vi "Caja fuerte No muerta.vi"() -> ()   [LabVIEW 2022 SP3]
doc: "Mi caja fuerte por Vess:3\n\nsimula el movimiento de una caja fuerte a la cual hay que darle una combinación y ya con esta saber\nsi la combinación es correcta o mala y después usar producto consumidor para enlistar los datos que van\na ser los movimientos que se harán para simular que la perilla gire"
panel:
  in  "Manija":i32(knob) min=0 max=100 step=1 scale=0.0..30.0
  out "Mensaje":string
  out "Arreglo C.":i32[](array[numeric])
  in  "Reinicio":bool
  in  "Enum":T1(ring)
  in  "stop":bool
  # "Combinación:\n11-7-10-21"
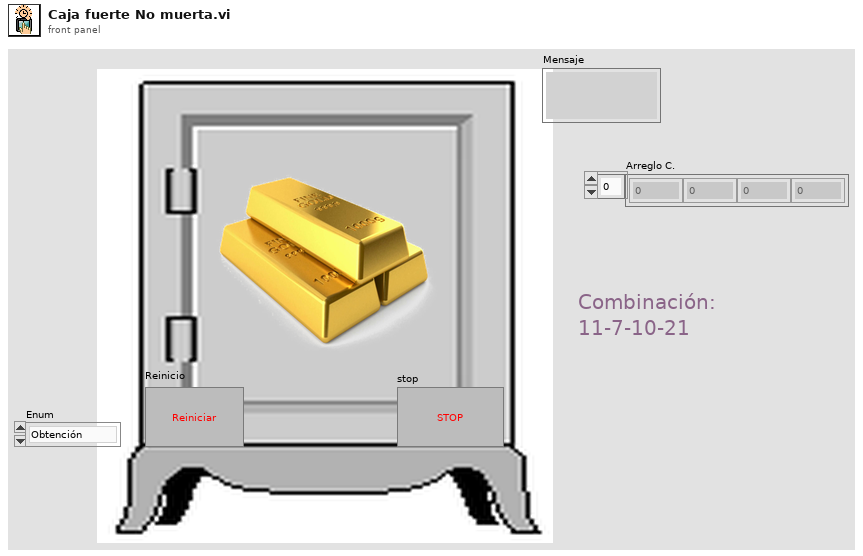
[diagram p1: front panel]
types:
  T1 = enum16{"Obtención", "Comprobación", "Fallo ", "Logro"}
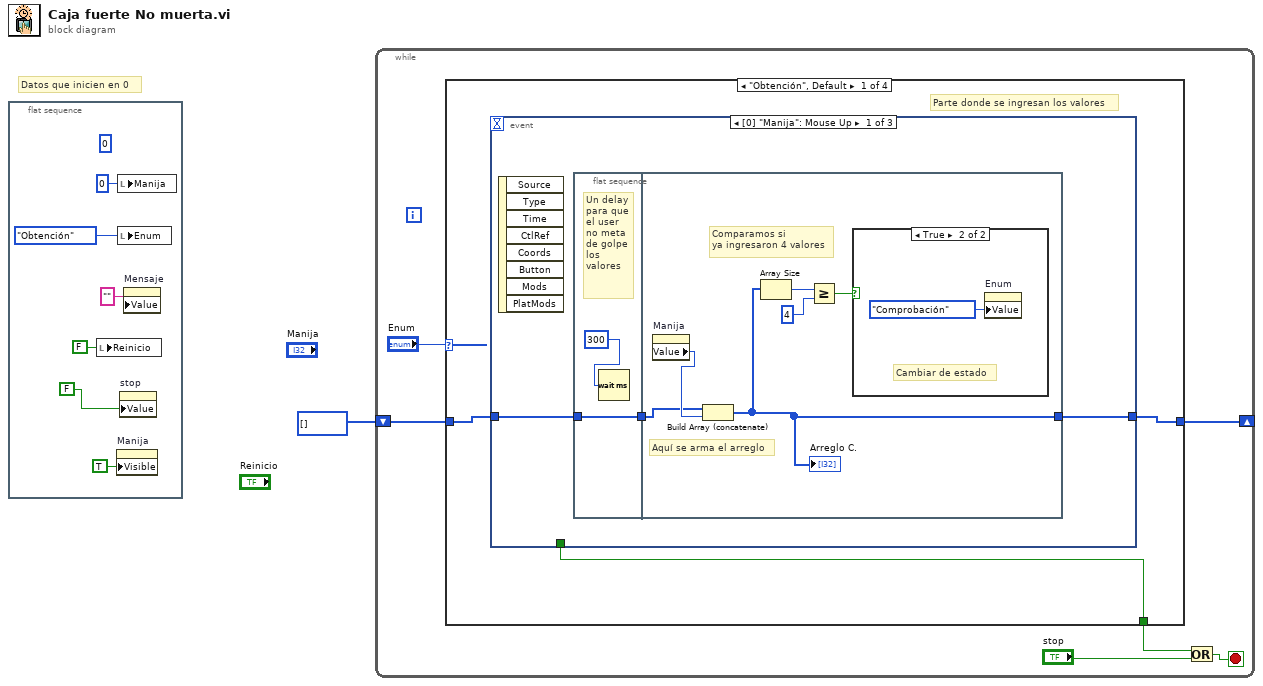
[diagram p0: block diagram]
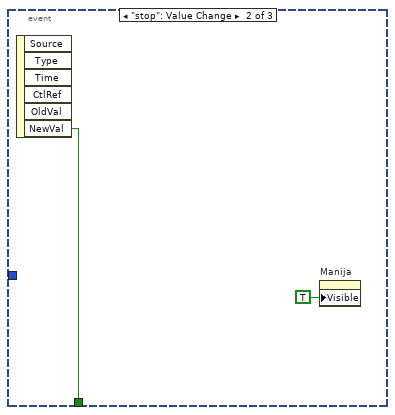
[diagram p3: hidden frame]
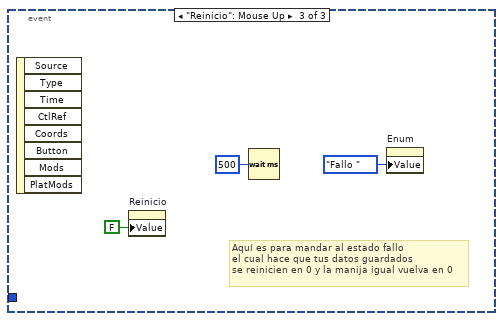
[diagram p4: hidden frame]
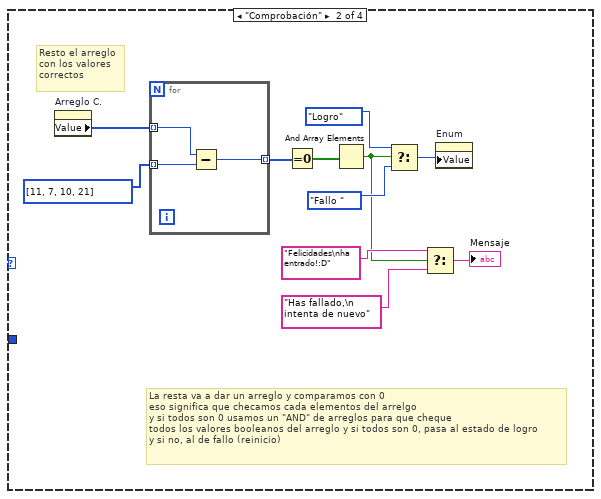
[diagram p5: hidden frame]
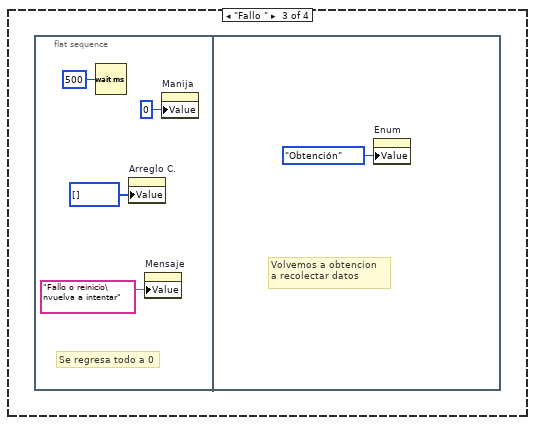
[diagram p6: hidden frame]
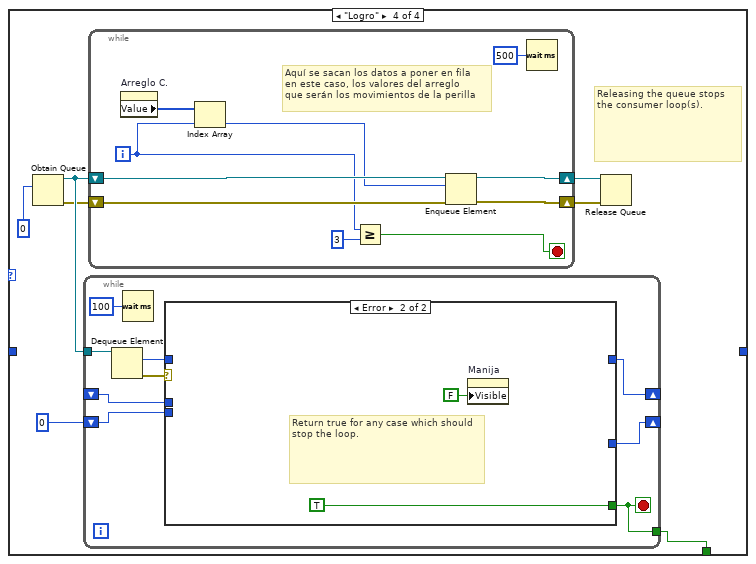
[diagram p7: hidden frame]
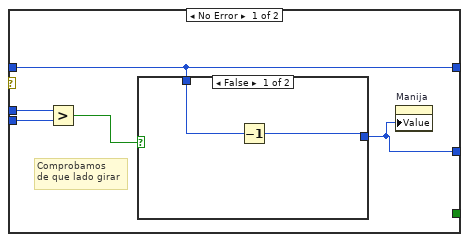
[diagram p8: hidden frame]
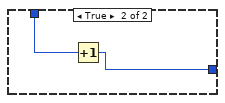
[diagram p9: hidden frame]
diagram:
  # "Datos que inicien en 0"
  n1 = flat-sequence {
    frame #0 {
      (unwired) 0 ("Manija")
      n2 = local write "Reinicio"(FALSE ("Reinicio")) -> ()
      n3 = property on="Manija" class="Knob (strict)"("Visible"=TRUE) -> ()  [unwired: 2 in, 2 out]
      n4 = local write "Manija"(0 ("Manija")) -> ()
      n5 = local write "Enum"(T1."Obtención" ("Enum")) -> ()
      n6 = property on="stop" class="Bool (strict)"("Value"=FALSE ("stop")) -> ()  [unwired: 2 in, 2 out]
      n7 = property on="Mensaje" class="Str"("Value"="" ("Mensaje")) -> ()  [unwired: 2 in, 2 out]
    }
  }
  n8 = while {
    shift-right: [w9] -> _
    shift-left: i32[] [] -> [w8]
    stop <- w10 stop-if-true
    n9 = case shown="\"Obtención\", Default" "Enum" {
      tunnel: [w16 _ _ w53] -> w12
      tunnel: w8 -> [w15 _ _ _]
      tunnel: [w14 _ _ _] -> w9
      frame "Obtención", Default {
        # "Parte donde se ingresan los valores"
        n10 = event shown="[0] \"Manija\": Mouse Up" {
          selector: _ -> [_ _ _]
          dyn-events: _ -> [_ _ _]
          timeout: _ -> [_ _ _]
          tunnel: [_ w30 _] -> w16
          tunnel: w15 -> [w19 _ _]
          tunnel: [w17 _ _] -> w14
          event "Manija": Mouse Up {
            n11 = event-data() -> ()  [unwired: 1 in, 8 out]
            n12 = flat-sequence {
              tunnel: w19 -> [w20]
              tunnel: [w20] -> w18
              tunnel: w18 -> [w23]
              tunnel: [w22] -> w17
              frame #0 {
                # "Un delay\npara que\nel user\nno meta\nde golpe\nlos \nvalores"
                n13 = Wait (ms)(milliseconds to wait=300) -> ()  [unwired: 1 out]
              }
              frame #1 {
                # "Comparamos si\nya ingresaron 4 valores"
                # "Aquí se arma el arreglo"
                n14 = property on="Manija" class="Knob (strict)"() -> ("Value"=w24:i32)  [unwired: 2 in, 2 out]
                n15 = Build Array (concatenate)(w23, w24) -> (w22:i32[])
                "Arreglo C." <- w22
                n16 = Array Size(array=w22) -> (size(s)=w27:i32)
                n17 = Greater Or Equal?(x=w27, y=4) -> (x >= y?=w25:bool)
                n18 = case shown="True" w25 {
                  frame False {
                  }
                  frame True {
                    # "Cambiar de estado"
                    n19 = property on="Enum" class="Enum (strict)"("Value"=T1."Comprobación" ("Enum")) -> ()  [unwired: 2 in, 2 out]
                  }
                }
              }
            }
          }
          event "stop": Value Change {
            n20 = event-data() -> ("NewVal"=w30:bool)  [unwired: 1 in, 5 out]
            n21 = property on="Manija" class="Knob (strict)"("Visible"=TRUE) -> ()  [unwired: 2 in, 2 out]
          }
          event "Reinicio": Mouse Up {
            # "Aquí es para mandar al estado fallo \nel cual hace que tus datos guardados \nse reinicien en 0 y la manija igual vuelva en 0"
            n22 = event-data() -> ()  [unwired: 1 in, 8 out]
            n23 = property on="Reinicio" class="Bool (strict)"("Value"=FALSE ("Reinicio")) -> ()  [unwired: 2 in, 2 out]
            n24 = Wait (ms)(milliseconds to wait=u32 500) -> ()  [unwired: 1 out]
            n25 = property on="Enum" class="Enum (strict)"("Value"=T1."Fallo " ("Enum")) -> ()  [unwired: 2 in, 2 out]
          }
        }
      }
      frame "Comprobación" {
        # "La resta va a dar un arreglo y comparamos con 0\neso significa que checamos cada elementos del arrelgo\ny si todos son 0 usamos un \"AND\" de arreglos para que cheque\ntodos los valores booleanos del arreglo y si todos son 0, pasa al estado de logro\ny si no, al de fallo (reinicio)"
        # "Resto el arreglo \ncon los valores \ncorrectos"
        n26 = property on="Arreglo C." class="Arr (strict)"() -> ("Value"=w43:i32[])  [unwired: 2 in, 2 out]
        n27 = for {
          tunnel: i32[] [11, 7, 10, 21] -> [w47] mode=indexing
          tunnel: w43 -> [w46] mode=indexing
          tunnel: [w45] -> w42 mode=indexing
          n28 = Subtract(x=w46, y=w47) -> (x-y=w45:i32)
        }
        n29 = Equal To 0?(x=w42) -> (x = 0?=w41:bool[])
        n30 = And Array Elements(Boolean array=w41) -> (logical AND=w34:bool)
        n31 = Select(t=T1."Logro" ("Enum"), s=w34, f=T1."Fallo " ("Enum")) -> (s? t:f=w38:T1)
        n32 = Select(t="Felicidades\nha entrado!:D", s=w34, f="Has fallado,\n intenta de nuevo") -> (s? t:f=→"Mensaje":string)
        n33 = property on="Enum" class="Enum (strict)"("Value"=w38) -> ()  [unwired: 2 in, 2 out]
      }
      frame "Fallo " {
        n34 = flat-sequence {
          frame #0 {
            # "Se regresa todo a 0"
            n35 = Wait (ms)(milliseconds to wait=u32 500) -> ()  [unwired: 1 out]
            n36 = property on="Arreglo C." class="Arr (strict)"("Value"=i32[] [] ("Arreglo C.")) -> ()  [unwired: 2 in, 2 out]
            n37 = property on="Mensaje" class="Str"("Value"="Fallo o reinicio\nvuelva a intentar" ("Mensaje")) -> ()  [unwired: 2 in, 2 out]
            n38 = property on="Manija" class="Knob (strict)"("Value"=0 ("Manija")) -> ()  [unwired: 2 in, 2 out]
          }
          frame #1 {
            # "Volvemos a obtencion\na recolectar datos"
            n39 = property on="Enum" class="Enum (strict)"("Value"=T1."Obtención" ("Enum")) -> ()  [unwired: 2 in, 2 out]
          }
        }
      }
      frame "Logro" {
        # "Releasing the queue stops the consumer loop(s)."
        n40 = Obtain Queue(element data type=0) -> (queue out=w59:refnum<queue>, error out=w58:errorcluster)  [unwired: 4 in, 1 out]
        n41 = while {
          tunnel: w59 -> [w78]
          shift-right: [w75] -> _
          shift-left: _ -> [w74]
          shift-right: [w72] -> _
          shift-left: 0 ("Manija") -> [w73]
          tunnel: [w71] -> w53
          stop <- w71 stop-if-true
          n42 = Dequeue Element(queue=w78) -> (element=w76:i32, error out=w77:errorcluster)  [unwired: 2 in, 2 out]
          n43 = Wait (ms)(milliseconds to wait=u32 100) -> ()  [unwired: 1 out]
          n44 = case shown="Error" w77 {
            tunnel: w76 -> [w80 _]
            tunnel: [_ TRUE] -> w71
            tunnel: [w80 _] -> w75
            tunnel: w74 -> [w83 _]
            tunnel: w73 -> [w82 _]
            tunnel: [w79 _] -> w72
            frame No Error {
              # "Comprobamos\nde que lado girar"
              n45 = Greater?(x=w83, y=w82) -> (0:w81:bool)
              n46 = case shown="False" w81 {
                tunnel: w80 -> [w85 w87]
                tunnel: [w84 w86] -> w79
                frame False {
                  n47 = Decrement(x=w85) -> (x-1=w84:i32)
                }
                frame True {
                  n48 = Increment(x=w87) -> (x+1=w86:i32)
                }
              }
              n49 = property on="Manija" class="Knob (strict)"("Value"=w79) -> ()  [unwired: 2 in, 2 out]
            }
            frame Error {
              # "Return true for any case which should stop the loop."
              n50 = property on="Manija" class="Knob (strict)"("Visible"=FALSE) -> ()  [unwired: 2 in, 2 out]
            }
          }
        }
        n51 = while {
          shift-right: [w67] -> w56
          shift-left: w58 -> [w68]
          shift-right: [w69] -> w57
          shift-left: w59 -> [w65]
          i -> [w62]
          stop <- w60 stop-if-true
          # "Aquí se sacan los datos a poner en fila\nen este caso, los valores del arreglo\nque serán los movimientos de la perilla"
          n52 = property on="Arreglo C." class="Arr (strict)"() -> ("Value"=w64:i32[])  [unwired: 2 in, 2 out]
          n53 = Index Array(array=w64, index=w62) -> (element=w63:i32)
          n54 = Greater Or Equal?(x=w62, y=3) -> (x >= y?=w60:bool)
          n55 = Enqueue Element(queue=w65, element=w63, error in (no error)=w68) -> (queue out=w69:refnum<queue>, error out=w67:errorcluster)  [unwired: 1 in, 1 out]
          n56 = Wait (ms)(milliseconds to wait=u32 500) -> ()  [unwired: 1 out]
        }
        n57 = Release Queue(queue=w57, error in (no error)=w56) -> ()  [unwired: 1 in, 3 out]
      }
    }
    n58 = Or(x=w12, y="stop") -> (x .or. y?=w10:bool)
  }
